vi "step4 TestIfUpperCrossSolvedSolved.vi"(8 "error in (no error)":errorcluster, 11 "cube in":T1) -> (0 "error out":errorcluster, 2 "upper cross solved?":bool)   [LabVIEW 2011]
uses:
  Typedef/cube.ctl
  Typedef/face.ctl
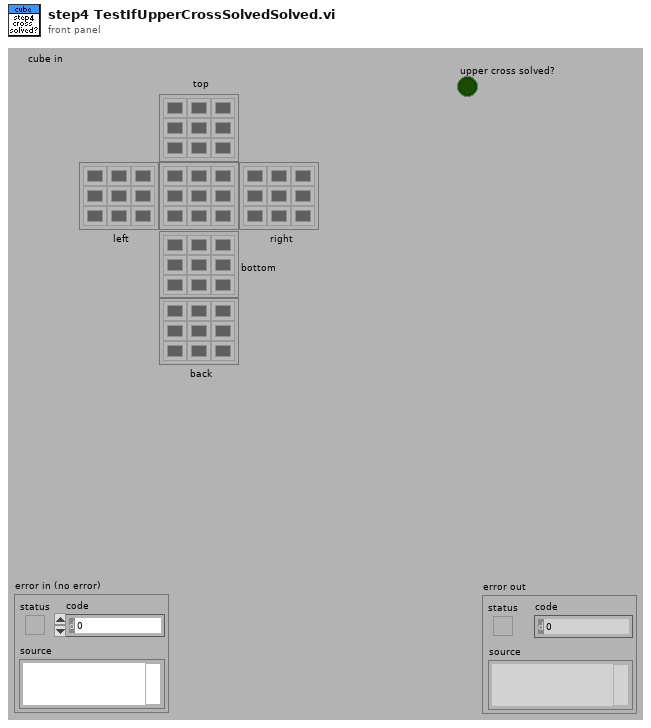
[diagram p1: front panel]
types:
  T1 = typedef "cube.ctl" = cluster{"top":T2, "left":T2, "right":T2, "bottom":T2, "back":T2, "front":T2}
  T2 = typedef "face.ctl" = u32[][]
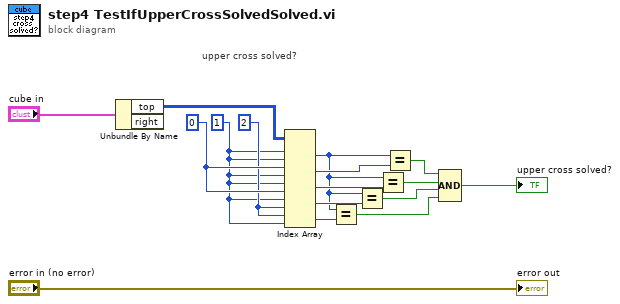
[diagram p0: block diagram]
diagram:
  w10 = 2 ("index (row)")
  w9 = 1 ("index (row)")
  w11 = 0 ("index (row)")
  # "upper cross solved?"
  n1 = Unbundle By Name("cube in") -> ("top"=w14:T2)  [unwired: 1 out]
  n2 = Index Array(array=w14, index (row) #1=w9, index (col) #1=w9, index (row) #2=w11, index (col) #2=w9, index (row) #3=w9, index (col) #3=w11, index (row) #4=w9, index (col) #4=w10, index (row) #5=w10, index (col) #5=w9) -> (element #1=w6:u32, element #2=w13:u32, element #3=w8:u32, element #4=w7:u32, element #5=w5:u32)
  n3 = Equal?(x=w6, y=w5) -> (x = y?=w2:bool)
  n4 = Equal?(x=w6, y=w7) -> (x = y?=w3:bool)
  n5 = Equal?(x=w6, y=w8) -> (x = y?=w4:bool)
  n6 = Equal?(x=w6, y=w13) -> (x = y?=w12:bool)
  n7 = Compound Arithmetic op=AND(w12, w4, w3, w2) -> (→"upper cross solved?":bool)
  "error out" <- "error in (no error)"
